vi "InitPH_AnyThread.vi"(10 "mode":T2 items=["Histo"=0, "T2"=2, "T3"=3], 11 "Library Version":string="3.0") -> (0 "Error":errorcluster, 2 "Init Info":T1, 3 "DevIdx":i32)   [LabVIEW 2017]
uses:
  PH_MeasMode.ctl
  PH_InitInfo.ctl
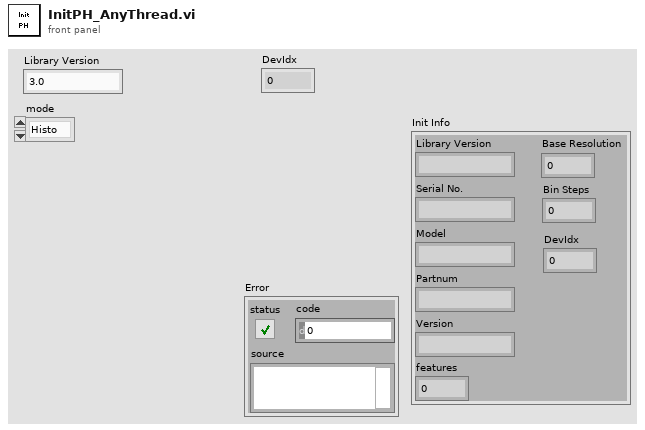
[diagram p1: front panel]
types:
  T1 = typedef "PH_InitInfo.ctl" = cluster{"Library Version":string, "Serial No.":string, "Model":string, "Partnum":string, "Version":string, "features":i32, "Base Resolution":dbl, "Bin Steps":i32, "DevIdx":i32}
  T2 = typedef "PH_MeasMode.ctl" = i32
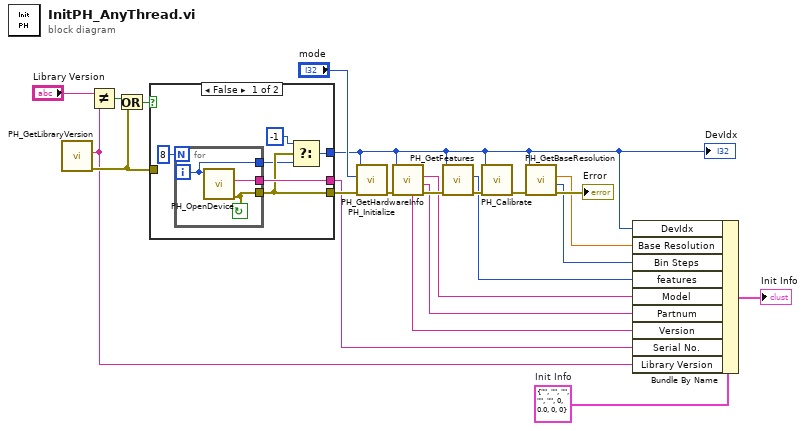
[diagram p0: block diagram]
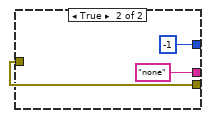
[diagram p2: hidden frame]
diagram:
  w11 = T1 {"Library Version"="", "Serial No."="", "Model"="", "Partnum"="", "Version"="", "features"=0, "Base Resolution"=0.0, "Bin Steps"=0, "DevIdx"=0}  # Init Info
  n1 = call "PH_GetLibraryVersion.vi"() -> ("error out"=w19:errorcluster, "Version"=w3:string)  [unwired: 9 in, 1 out]
  n2 = Not Equal?(x="Library Version", y=w3) -> (x != y?=w20:bool)
  n3 = Or(x=w20, y=w19) -> (x .or. y?=w21:bool)
  n4 = case shown="False" w21 {
    tunnel: [w24 -1 ("return type")] -> w1
    tunnel: [w27 "none" ("serial")] -> w4
    tunnel: [w26 w32] -> w18
    tunnel: w19 -> [_ w32]
    frame False {
      n5 = for {
        N: 8 -> [_]
        tunnel: [w31] -> w26
        tunnel: [w30] -> w27
        tunnel: [w29] -> w25
        i -> [w29]
        stop <- w31 continue-if-true
        n6 = call "PH_OpenDevice.vi"("devidx"=w29) -> ("error out"=w31:errorcluster, "serial"=w30:string)  [unwired: 8 in, 1 out]
      }
      n7 = Select(t=-1, s=w26, f=w25) -> (s? t:f=w24:i32)
    }
    frame True {
    }
  }
  "DevIdx" <- w1
  n8 = call "PH_Initialize.vi"("error in (no error)"=w18, "mode"="mode", "devidx"=w1) -> ("error out"=w16:errorcluster)  [unwired: 7 in, 1 out]
  n9 = call "PH_GetHardwareInfo.vi"("error in (no error)"=w16, "devidx"=w1) -> ("error out"=w15:errorcluster, "Partnum"=w6:string, "Model"=w7:string, "Version"=w5:string)  [unwired: 5 in, 1 out]
  n10 = call "PH_GetFeatures.vi"("error in (no error)"=w15, "devidx"=w1) -> ("error out"=w14:errorcluster, "features"=w8:i32)  [unwired: 7 in, 1 out]
  n11 = call "PH_Calibrate.vi"("error in (no error)"=w14, "devidx"=w1) -> ("error out"=w13:errorcluster)  [unwired: 8 in, 1 out]
  n12 = call "PH_GetBaseResolution.vi"("error in (no error)"=w13, "devidx"=w1) -> ("error out"=→"Error":errorcluster, "binsteps"=w9:i32, "resolution"=w10:dbl)  [unwired: 6 in, 1 out]
  n13 = Bundle By Name(cluster=w11, "DevIdx"=w1, "Base Resolution"=w10, "Bin Steps"=w9, "features"=w8, "Model"=w7, "Partnum"=w6, "Version"=w5, "Serial No."=w4, "Library Version"=w3) -> (→"Init Info":T1)
